vi "未命名 1.vi"() -> ()   [LabVIEW 2012]
panel:
  in  "布尔":bool
  out "new picture":picture caption="新图片"
  in  "min distance":dbl=4200.0
  in  "max distance":dbl=4200.0
  in  "distance":dbl=4200.0
  in  "point(x,y)":cluster{"x":i16, "y":i16} caption="点(x,y)"
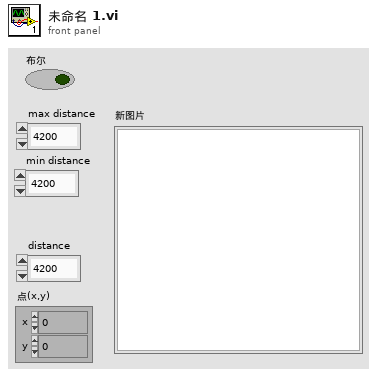
[diagram p1: front panel]
types:
  T1 = cluster{"Width":u16, "Style":enum32{"Solid", "Dash", "Dot", "DashDot", "DashDotDot"}}
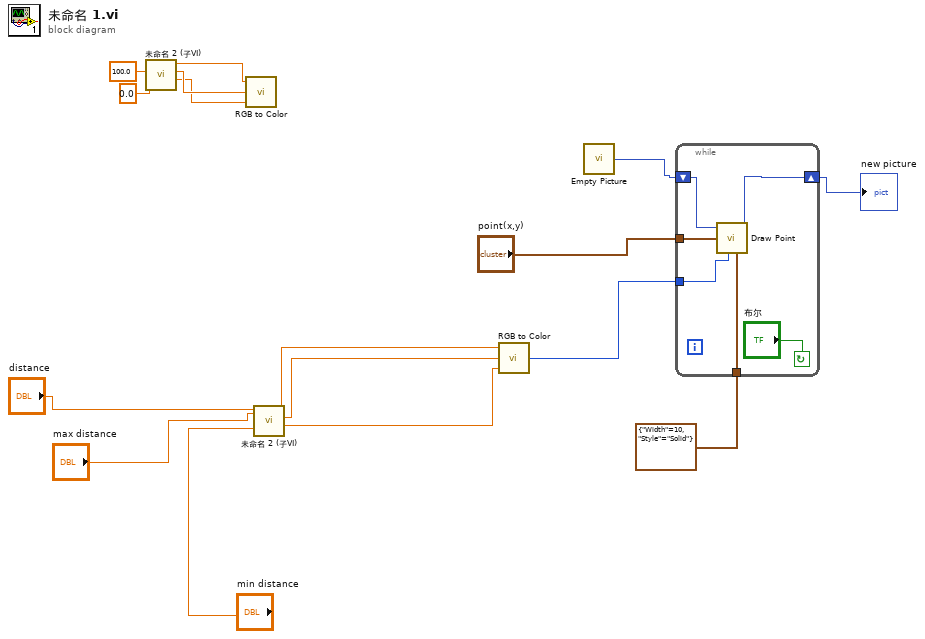
[diagram p0: block diagram]
diagram:
  n1 = call "未命名 2 (子VI).vi"("min distance"=0.0, "max distance"=100.0) -> ("b"=w3:dbl, "g"=w4:dbl, "r"=w5:dbl)  [unwired: 7 in]
  n2 = call <vilib>:"RGB to Color.vi"("B"=w3, "G"=w4, "R"=w5) -> ()  [unwired: 1 out]
  n3 = call "未命名 2 (子VI).vi"("min distance"="min distance", "max distance"="max distance", "distance"="distance") -> ("b"=w11:dbl, "g"=w12:dbl, "r"=w13:dbl)  [unwired: 6 in]
  n4 = call <vilib>:"RGB to Color.vi"("B"=w11, "G"=w12, "R"=w13) -> ("Color"=w14:u32)
  n5 = call "Empty Picture"() -> ("empty picture"=w2:picture)
  n6 = while {
    tunnel: "point(x,y)" -> [w22]
    tunnel: T1 {"Width"=10, "Style"=enum."Solid"} ("pen") -> [w21]
    tunnel: w14 -> [w20]
    shift-right: [w18] -> w1
    shift-left: w2 -> [w19]
    stop <- "布尔" continue-if-true
    n7 = call <vilib>:"Draw Point.vi"("picture"=w19, "point(x,y)"=w22, "color(black)"=w20, "pen"=w21) -> ("new picture"=w18:picture)  [unwired: 5 in]
  }
  "new picture" <- w1
